vi "Query Marker.vi"(8 "error in (no error)":errorcluster, 10 "Active Marker (1: Marker1)":i32(ring)=1 items=["Marker1"=1, "Marker2"=2, "Marker3"=3, "Marker4"=4, "Marker5"=5, "Marker6"=6, "Marker7"=7, "Marker8"=8, "Marker9"=9, "Marker10"=10, "Marker11"=11, "Marker12"=12], 11 "VISA resource name":refnum<visa-resource-name>) -> (0 "error out":errorcluster, 1 "Marker Amplitude":dbl, 2 "Marker Position":dbl, 3 "VISA resource name out":refnum<visa-resource-name>)   [LabVIEW 2018, in "Agilent MXA Series.lvlib"]
doc: "Returns the x-position and amplitude of a specified marker."
uses:
  Agilent MXA Series.lvlib
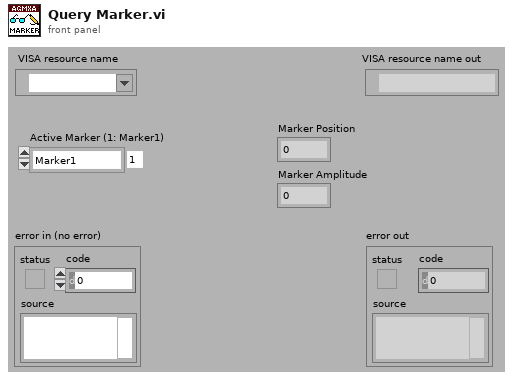
[diagram p1: front panel]
types:
  T1 = typedef "Agilent MXA Series.lvlib/Extended User Data.ctl" = cluster{"Measurement Type":i32, "Agilent MXA/EXA Model":i32}
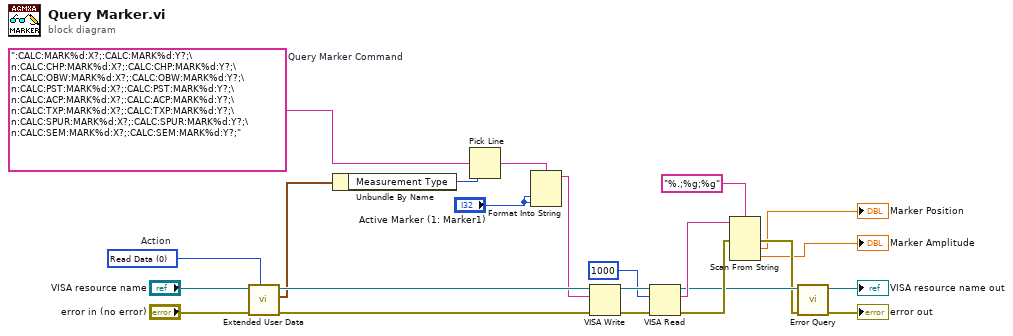
[diagram p0: block diagram]
diagram:
  w6 = ":CALC:MARK%d:X?;:CALC:MARK%d:Y?;\n:CALC:CHP:MARK%d:X?;:CALC:CHP:MARK%d:Y?;\n:CALC:OBW:MARK%d:X?;:CALC:OBW:MARK%d:Y?;\n:CALC:PST:MARK%d:X?;:CALC:PST:MARK%d:Y?;\n:CALC:ACP:MARK%d:X?;:CALC:ACP:MARK%d:Y?;\n:CALC:TXP:MARK%d:X?;:CALC:TXP:MARK%d:Y?;\n:CALC:SPUR:MARK%d:X?;:CALC:SPUR:MARK%d:Y?;\n:CALC:SEM:MARK%d:X?;:CALC:SEM:MARK%d:Y?;"  # Query Marker Command
  w11 = 0 items=["Read Data", "Write Data", "Clear Data", "Clear ALL Data"]  # Action
  n1 = call "Extended User Data.vi"("Action (1:Write Data)"=w11, "Error In (no error)"="error in (no error)", "VISA resource name in"="VISA resource name") -> ("Error Out"=w9:errorcluster, "User Data Out"=w8:T1, "VISA resource name out"=w10:refnum<visa-resource-name>)  [unwired: 6 in]
  n2 = Unbundle By Name(w8) -> ("Measurement Type"=w7:i32)
  n3 = Pick Line(multi-line string=w6, line index=w7) -> (output string=w4:string)  [unwired: 1 in]
  n4 = Format Into String(format string=w4, "Active Marker (1: Marker1)", "Active Marker (1: Marker1)") -> (resulting string=w3:string)  [unwired: 2 in, 1 out]
  n5 = VISA Write(VISA resource name=w10, write buffer=w3, error in (no error)=w9) -> (VISA resource name out=w22:refnum<visa-resource-name>, error out=w23:errorcluster)  [unwired: 1 out]
  n6 = VISA Read(VISA resource name=w22, byte count=1000, error in (no error)=w23) -> (VISA resource name out=w17:refnum<visa-resource-name>, read buffer=w19:string, error out=w20:errorcluster)  [unwired: 1 out]
  n7 = Scan From String(format string="%.;%g;%g", input string=w19, error in=w20) -> (error out=w16:errorcluster, output 1=→"Marker Position":dbl, output 2=→"Marker Amplitude":dbl)  [unwired: 3 in, 2 out]
  n8 = call "Error Query.vi"("error in (no error)"=w16, "VISA resource name"=w17) -> ("error out"=→"error out":errorcluster, "VISA resource name out"=→"VISA resource name out":refnum<visa-resource-name>)  [unwired: 6 in, 2 out]
